vi "Get DoubleArray.vi"(8 "error in (no error)":errorcluster, 11 "DblArrayMsg In":refnum<class "DblArrayMsg.lvclass">) -> (0 "error out":errorcluster, 2 "Message Data":dbl[](array[numeric]), 3 "DblArrayMsg Out":refnum<class "DblArrayMsg.lvclass">)   [LabVIEW 2009, in "LapDog.Messaging.v2.NativeArrays.lvlib" / "DblArrayMsg.lvclass"]
doc: "Returns the data contained in the message.\n\nThis method executes regardless of the error in state."
uses:
  DblArrayMsg.lvclass
  DblArrayMsg.lvclass/DblArrayMsg.ctl
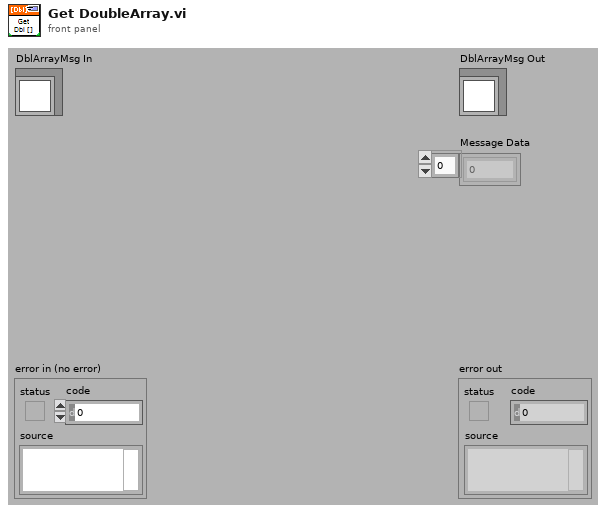
[diagram p1: front panel]
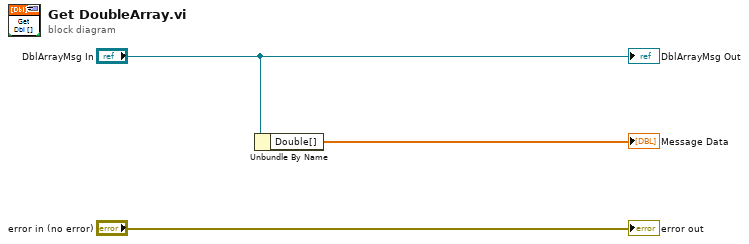
[diagram p0: block diagram]
diagram:
  n1 = Unbundle By Name("DblArrayMsg In") -> ("Double[]"=→"Message Data":dbl[])
  "error out" <- "error in (no error)"
  "DblArrayMsg Out" <- "DblArrayMsg In"
